vi "MDAQ_SurfaceSum.vi"(9 "Cluster IN":T1 {"CV"."Temperature Array" scale=0.0..100.0}, 10 "Status_Cluster IN":T3 {"GATESTOP" format="%04x"; "GATESTRT" format="%04x"; "AMPLITUDE" format="%04x"; "M_CYCLES" format="%04x"; "N_CYCLES" format="%04x"; "STEP" format="%04x"; "BASE" format="%04x"; "CHAN" format="%04x"}) -> (1 "Cluster Out":T1 {"CV"."Temperature Array" scale=0.0..100.0}, 2 "Status_Cluster Out":T3 {"GATESTOP" format="%04x"; "GATESTRT" format="%04x"; "AMPLITUDE" format="%04x"; "M_CYCLES" format="%04x"; "N_CYCLES" format="%04x"; "STEP" format="%04x"; "BASE" format="%04x"; "CHAN" format="%04x"}, 3 "CV.SurfaceCV":dbl[][](array[numeric]))   [LabVIEW 2021]
uses:
  Status_Cluster.ctl
  GUI_Def.ctl
  Mode_Enum.ctl
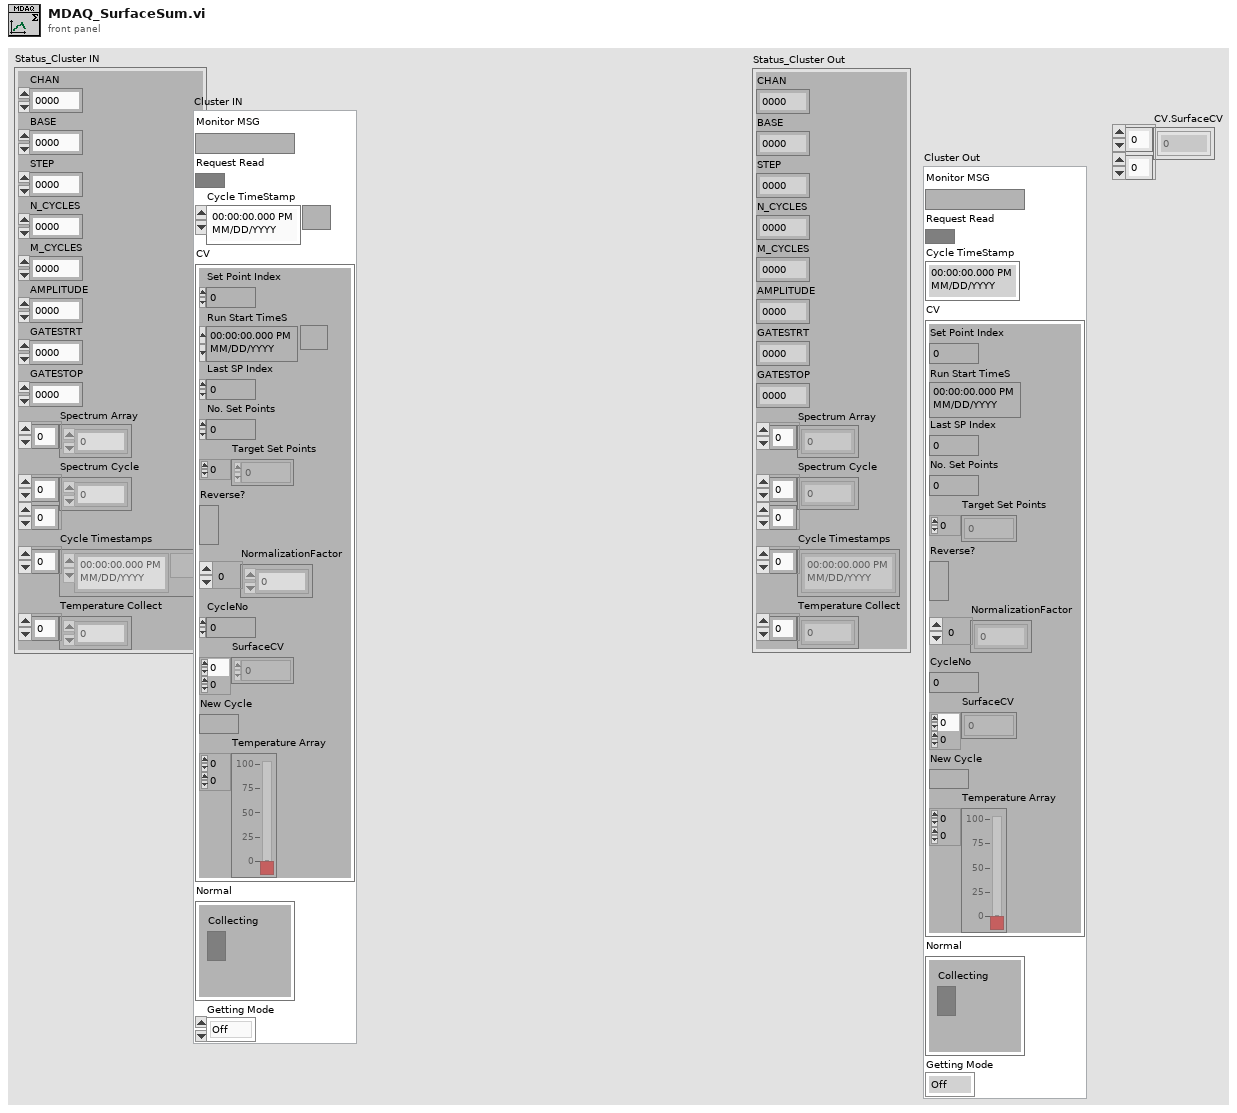
[diagram p1: front panel]
types:
  T1 = typedef "GUI_Def.ctl" = cluster{"Monitor MSG":string, "Request Read":bool, "Cycle TimeStamp":timestamp, "CV":cluster{"Set Point Index":u32, "Run Start TimeS":timestamp, "Last SP Index":u32, "No. Set Points":u32, "Target Set Points":i32[], "Reverse?":bool, "NormalizationFactor":i32[], "CycleNo":i32, "SurfaceCV":dbl[][], "New Cycle":bool, "Temperature Array":dbl[][]}, "Normal":cluster{"Collecting":bool}, "Getting Mode":T2}
  T2 = typedef "Mode_Enum.ctl" = enum16{"Off", "Normal", "CV+Temp", "CV"}
  T3 = typedef "Status_Cluster.ctl" = cluster{"CHAN":u32, "BASE":u32, "STEP":u32, "N_CYCLES":u32, "M_CYCLES":u32, "AMPLITUDE":u32, "GATESTRT":u32, "GATESTOP":u32, "Spectrum Array":u32[], "Spectrum Cycle":u32[][], "Cycle Timestamps":timestamp[], "Temperature Collect":dbl[]}
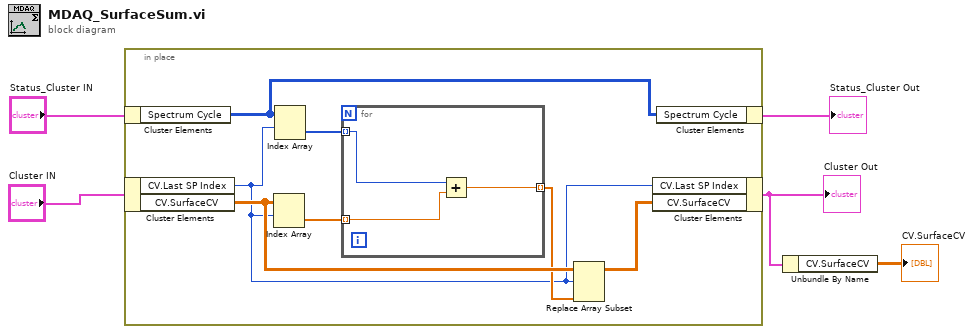
[diagram p0: block diagram]
diagram:
  n1 = in-place {
    n2 = in-place-cluster #1("Status_Cluster IN") -> ("Spectrum Cycle"=w6:u32[][])
    n3 = in-place-cluster #2("Cluster IN") -> ("CV.Last SP Index"=w7:u32, "CV.SurfaceCV"=w10:dbl[][])
    n4 = Index Array(array=w10, index (row)=w7) -> (element=w11:dbl[])  [unwired: 1 in]
    n5 = Index Array(array=w6, index (row)=w7) -> (element=w12:u32[])  [unwired: 1 in]
    n6 = for {
      tunnel: w12 -> [w15] mode=indexing
      tunnel: w11 -> [w14] mode=indexing
      tunnel: [w13] -> w9 mode=indexing
      n7 = Add(x=w15, y=w14) -> (x+y=w13:dbl)
    }
    n8 = Replace Array Subset(array=w10, new element=w9, index (row)=w7) -> (w8:dbl[][])  [unwired: 1 in]
    n9 = in-place-cluster #2("CV.Last SP Index"=w7, "CV.SurfaceCV"=w8) -> (w2:T1)
    n10 = in-place-cluster #1("Spectrum Cycle"=w6) -> (→"Status_Cluster Out":T3)
  }
  "Cluster Out" <- w2
  n11 = Unbundle By Name(w2) -> ("CV.SurfaceCV"=→"CV.SurfaceCV":dbl[][])
